vi "Set_Hi-Tec_server.vi"(4 "Client Name":string, 5 "Gas Line Name":T1, 6 "Strength (% by volume)":dbl min=0.0 max=1000.0 format="%.3f", 7 "Carrier_2 Q (l/min)":dbl=20.0 format="%.2f", 8 "Carrier_1 Q (l/min)":dbl=20.0 format="%.2f", 9 "Mode":enum16{"Control Hi-Tec", "Check Hi-Tec Demands"}(ring)) -> (0 "Flowrates (kg/min)":dbl[](array[numeric]) format="%.2f", 1 "Comment":string)   [LabVIEW 2022 SP3]
uses:
  Anemometry/Anemometry Sub Vis/Controls/GMU Gas Line Name.ctl
  ADAM Client/Sub VIs/ADAM Controls/Ch_description_ADAM.ctl
  ADAM Client/Sub VIs/ADAM Controls/Module_type_ADAM.ctl
  ADAM Client/Sub VIs/ADAM Controls/Function_ADAM.ctl
  ADAM Client/Sub VIs/ADAM Controls/Channel_State.ctl
  ADAM Client/Sub VIs/ADAM Controls/Calib_type_ADAM.ctl
  ADAM Client/Sub VIs/ADAM Controls/Address.ctl
  ADAM Client/Sub VIs/ADAM Controls/Update_scan_value.ctl
  Anemometry/Anemometry Sub Vis/Globals/Gas_management_global.vi
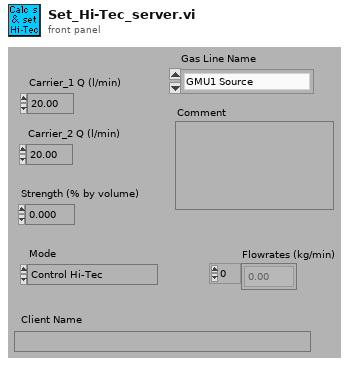
[diagram p1: front panel]
types:
  T1 = typedef "GMU Gas Line Name.ctl" = enum16{"GMU1 Source", "GMU2 Source", "GMU2 Calib", "CPP GRC-A", "CPP GRC-B"}
  T2 = typedef "Module_type_ADAM.ctl" = string
  T3 = typedef "Ch_description_ADAM.ctl" = cluster{"Ch Name":string, "Type":T2, "Function":T4, "Ch State":T5, "Calibration type":T6, "A":dbl, "B":dbl, "C":dbl, "D":dbl, "Comments":string, "Address":T7, "String":string, "Duty":u16}
  T4 = typedef "Function_ADAM.ctl" = enum16{"Analogue Input", "Digital Input", "Event counter", "Event rate", "Analogue Output", "Digital Output", "Relay Output"}
  T5 = typedef "Channel_State.ctl" = enum16{"On", "Off", "Always On", "Always Off"}
  T6 = typedef "Calib_type_ADAM.ctl" = string
  T7 = typedef "Address.ctl" = cluster{"Main":i32, "Ch.":i32, "Sub":i32, "Port Name":string}
  T8 = enum16{"Append to Global", "Read Global then Clear"}
  T9 = typedef "Update_scan_value.ctl" = cluster{"Channel Name":string, "New Value":dbl, "!Auto_Off":bool}
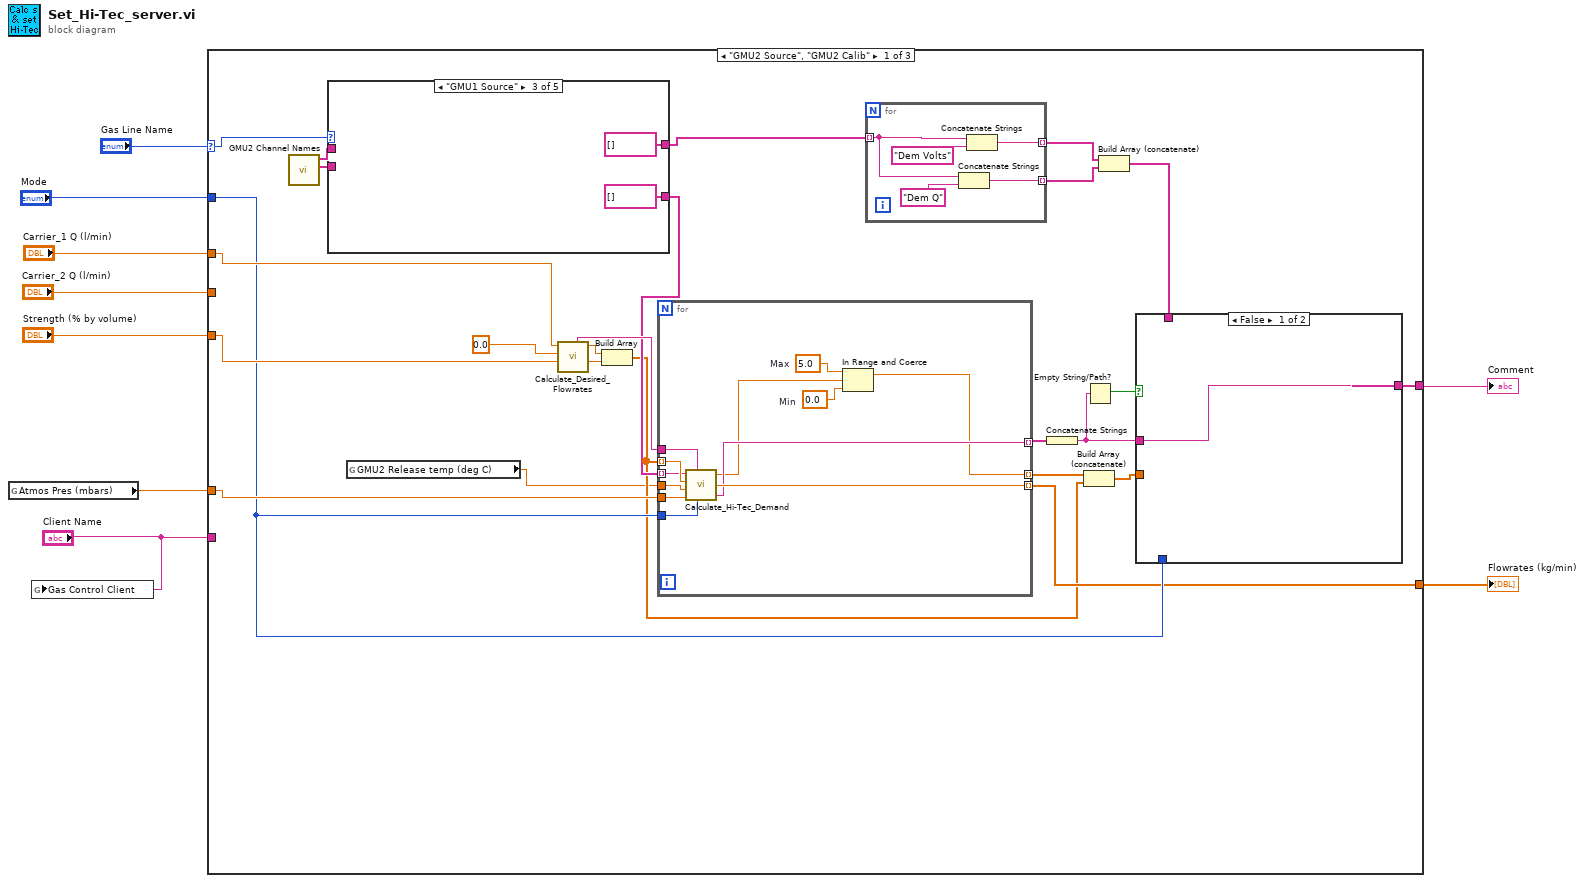
[diagram p0: block diagram]
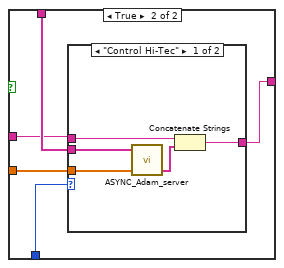
[diagram p2: hidden frame]
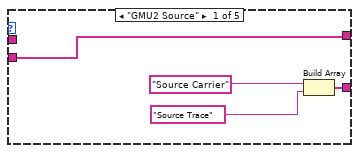
[diagram p4: hidden frame]
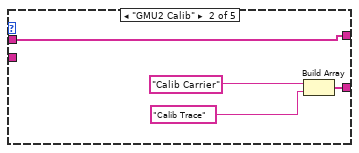
[diagram p5: hidden frame]
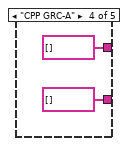
[diagram p6: hidden frame]
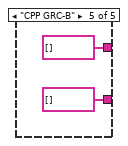
[diagram p7: hidden frame]
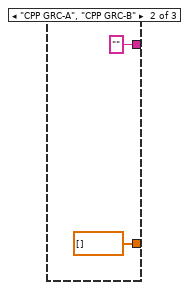
[diagram p8: hidden frame]
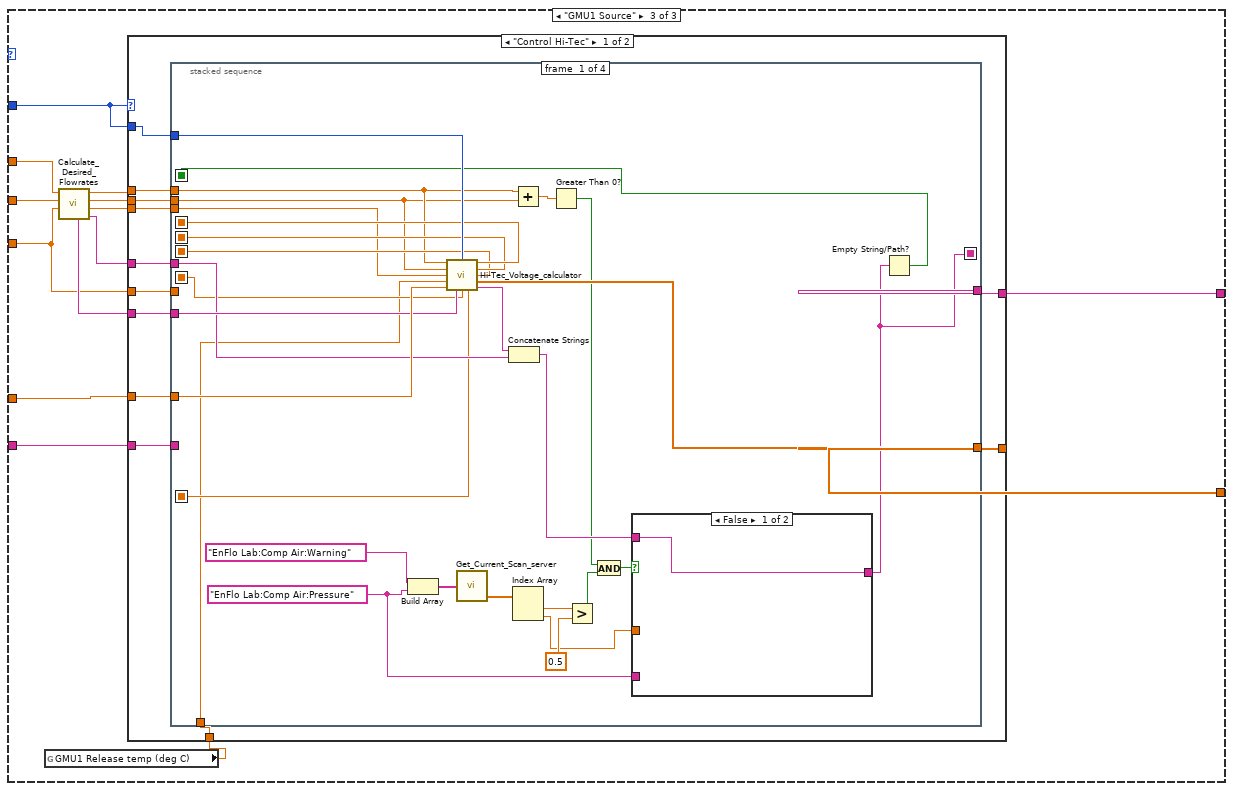
[diagram p9: hidden frame]
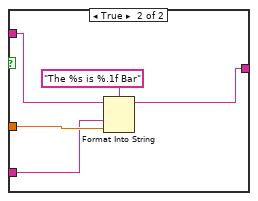
[diagram p10: hidden frame]
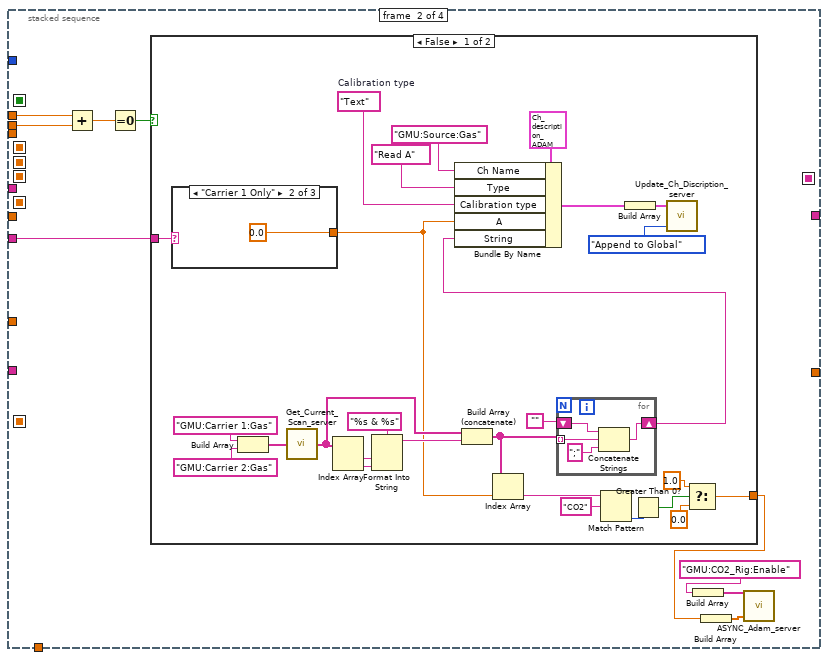
[diagram p11: hidden frame]
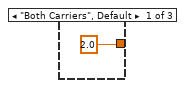
[diagram p12: hidden frame]
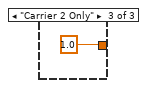
[diagram p13: hidden frame]
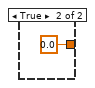
[diagram p14: hidden frame]
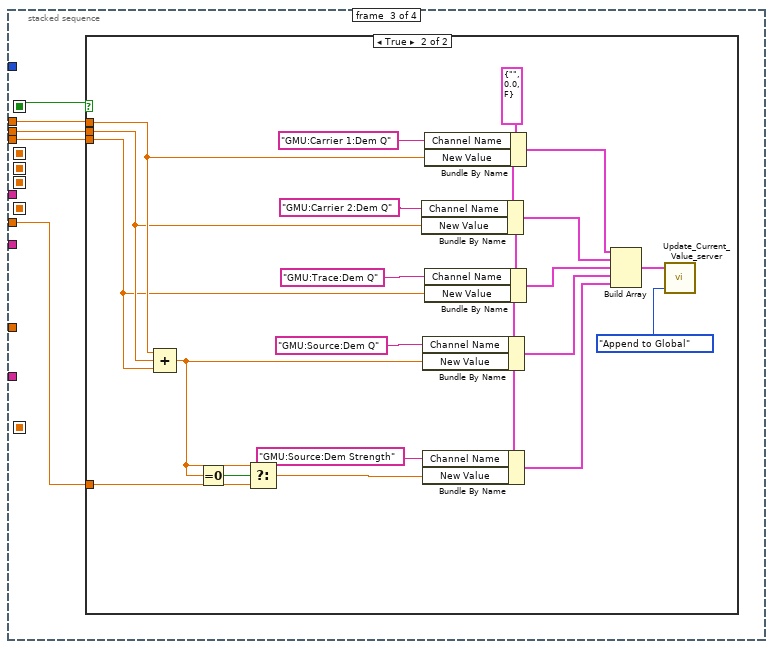
[diagram p15: hidden frame]
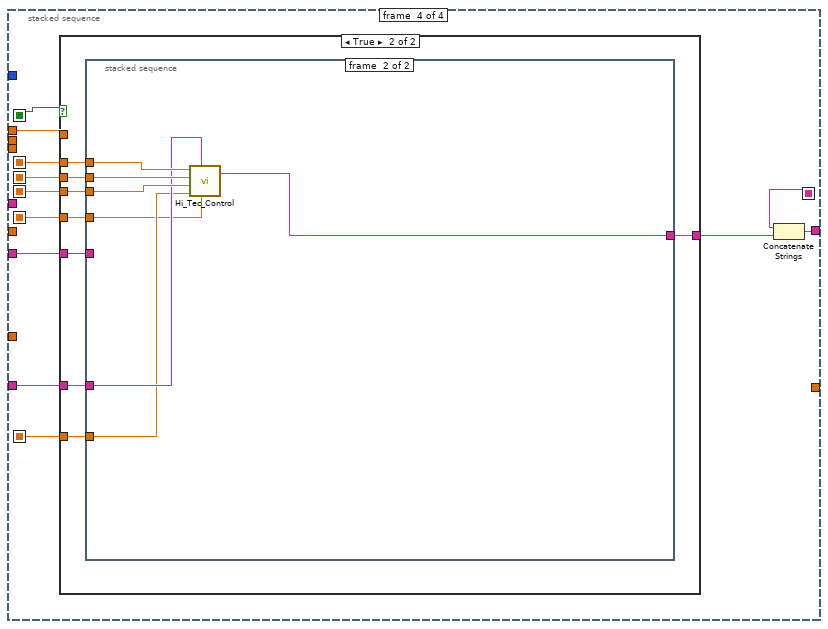
[diagram p17: hidden frame]
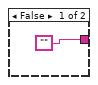
[diagram p18: hidden frame]
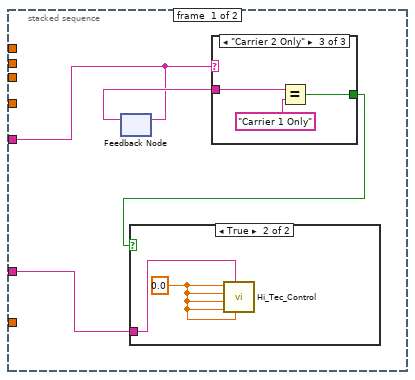
[diagram p19: hidden frame]
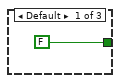
[diagram p20: hidden frame]
diagram:
  n1 = global read "Gas_management_global.vi" "Atmos Pres (mbars)"() -> (w9:dbl)
  n2 = global write "Gas_management_global.vi" "Gas Control Client"("Client Name") -> ()
  n3 = case shown="\"GMU2 Source\", \"GMU2 Calib\"" "Gas Line Name" {
    selector: "Gas Line Name" -> [w27 _ _]
    tunnel: w9 -> [w26 _ w93]
    tunnel: [w24 dbl[] [] ("Flowrates (kg/min)") w92] -> w8
    tunnel: "Mode" -> [w25 _ w91]
    tunnel: "Client Name" -> [_ _ w90]
    tunnel: "Carrier_1 Q (l/min)" -> [w29 _ w89]
    tunnel: "Carrier_2 Q (l/min)" -> [_ _ w88]
    tunnel: "Strength (% by volume)" -> [w28 _ w83]
    tunnel: [w23 "" w81] -> w2
    frame "GMU2 Source", "GMU2 Calib" {
      n4 = call "GMU2 Channel Names.vi"() -> ("GMU2 Source Channels"=w18:string[], "GMU2 Calib Channels"=w11:string[])  [unwired: 10 in]
      n5 = case shown="\"GMU1 Source\"" w27 {
        tunnel: [w55 w59 string[] [] string[] [] string[] []] -> w30
        tunnel: [w52 w56 string[] [] string[] [] ("GMU2 Calib Channels") string[] [] ("GMU2 Calib Channels")] -> w19
        tunnel: w18 -> [w52 _ _ _ _]
        tunnel: w11 -> [_ w56 _ _ _]
        frame "GMU2 Source" {
          n6 = Build Array("Source Carrier", "Source Trace") -> (w55:string[])
        }
        frame "GMU2 Calib" {
          n7 = Build Array("Calib Carrier", "Calib Trace") -> (w59:string[])
        }
        frame "GMU1 Source" {
        }
        frame "CPP GRC-A" {
        }
        frame "CPP GRC-B" {
        }
      }
      n8 = global read "Gas_management_global.vi" "GMU2 Release temp (deg C)"() -> (w10:dbl)
      n9 = call "Calculate_Desired_Flowrates.vi"("Strength (% by volume)"=w28, "Carrier_2 Q (l/min)"=0.0, "Carrier_1 Q (l/min)"=w29) -> ("Trace Q l/min"=w33:dbl, "Carrier 1 l/min"=w34:dbl, "Carrier Info"=w32:string)  [unwired: 3 in, 2 out]
      n10 = Build Array(w34, w33) -> (w12:dbl[])
      n11 = for {
        tunnel: w26 -> [w77]
        tunnel: w10 -> [w76]
        tunnel: w12 -> [w75] mode=indexing
        tunnel: [w72] -> w24 mode=indexing
        tunnel: w30 -> [w74] mode=indexing
        tunnel: w32 -> [w73]
        tunnel: [w66] -> w14 mode=indexing
        tunnel: [w71] -> w22 mode=indexing
        tunnel: w25 -> [w70]
        w68 = 0.0  # Min
        w69 = 5.0  # Max
        n12 = call "Calculate_Hi-Tec_Demand.vi"("Gas Line Name"=w74, "Carrier Info"=w73, "Flowrate"=w75, "Release temp (deg C)"=w76, "Mode"=w70, "Atmos Pres (mbars)"=w77) -> ("Demand Voltage"=w67:dbl, "Flowrate (kg/min)"=w72:dbl, "Error messages"=w71:string)
        n13 = In Range and Coerce(upper limit=w69, x=w67, lower limit=w68) -> (coerced(x)=w66:dbl)  [unwired: 1 out]
      }
      n14 = for {
        tunnel: w19 -> [w37] mode=indexing
        tunnel: [w36] -> w17 mode=indexing
        tunnel: [w35] -> w16 mode=indexing
        n15 = Concatenate Strings(w37, "Dem Q" ("string")) -> (w35:string)
        n16 = Concatenate Strings(w37, "Dem Volts" ("string")) -> (w36:string)
      }
      n17 = Concatenate Strings(w22) -> (w21:string)
      n18 = Build Array (concatenate)(w14, w12) -> (w13:dbl[])
      n19 = Empty String/Path?(string/path=w21) -> (empty?=w20:bool)
      n20 = Build Array (concatenate)(w17, w16) -> (w15:string[])
      n21 = case shown="False" w20 {
        tunnel: w15 -> [_ w45]
        tunnel: w13 -> [_ w44]
        tunnel: w25 -> [_ w43]
        tunnel: [w40 w42] -> w23
        tunnel: w21 -> [w40 w41]
        frame False {
        }
        frame True {
          n22 = case shown="\"Control Hi-Tec\"" w43 {
            tunnel: w45 -> [w50 _]
            tunnel: w44 -> [w49 _]
            tunnel: w41 -> [w47 w51]
            tunnel: [w46 w51] -> w42
            frame "Control Hi-Tec" {
              n23 = call "ASYNC_Adam_server.vi"("Values"=w49, "Channel Names"=w50) -> ("Scan Comments"=w48:string[])  [unwired: 1 in, 2 out]
              n24 = Concatenate Strings(w47, w48) -> (w46:string)
            }
            frame "Check Hi-Tec Demands" {
            }
          }
        }
      }
    }
    frame "CPP GRC-A", "CPP GRC-B" {
    }
    frame "GMU1 Source" {
      n25 = global read "Gas_management_global.vi" "GMU1 Release temp (deg C)"() -> (w80:dbl)
      n26 = call "Calculate_Desired_Flowrates.vi"("Strength (% by volume)"=w83, "Carrier_2 Q (l/min)"=w88, "Carrier_1 Q (l/min)"=w89) -> ("Error Message"=w82:string, "Trace Q l/min"=w85:dbl, "Carrier 2 l/min"=w86:dbl, "Carrier 1 l/min"=w87:dbl, "Carrier Info"=w84:string)  [unwired: 3 in]
      n27 = case shown="\"Control Hi-Tec\"" w91 {
        tunnel: w87 -> [w105 w260]
        tunnel: w93 -> [w104 w261]
        tunnel: [w103 w253] -> w81
        tunnel: [w102 w259] -> w92
        tunnel: w91 -> [w101 w258]
        tunnel: w90 -> [w100 _]
        tunnel: w86 -> [w99 w257]
        tunnel: w85 -> [w98 w256]
        tunnel: w84 -> [w97 w255]
        tunnel: w83 -> [w96 _]
        tunnel: w82 -> [w95 w252]
        tunnel: w80 -> [w94 w251]
        frame "Control Hi-Tec" {
          n28 = stacked-sequence {
            seq-local: [w132 _ _ _] -> [_ _ w189 w217]
            seq-local: [w131 _ _ _] -> [_ _ _ w221]
            seq-local: [w130 _ _ _] -> [_ _ _ w220]
            seq-local: [w129 _ _ _] -> [_ _ _ w219]
            seq-local: [w116 _ _ _] -> [_ _ _ w214]
            seq-local: [w123 _ _ _] -> [_ _ _ w211]
            seq-local: [w122 _ _ _] -> [_ _ _ w210]
            tunnel: w99 -> [w112 w141 w187 _]
            tunnel: w105 -> [w113 w142 w188 w216]
            tunnel: w104 -> [w134 _ _ _]
            tunnel: [_ _ _ w215] -> w103
            tunnel: [w126 _ _ _] -> w102
            tunnel: w101 -> [w133 _ _ _]
            tunnel: w100 -> [_ _ _ w218]
            tunnel: w98 -> [w128 _ w186 _]
            tunnel: w97 -> [w127 w144 _ w212]
            tunnel: w96 -> [_ _ w185 _]
            tunnel: w95 -> [w124 _ _ _]
            tunnel: w94 -> [w106 _ _ _]
            frame #0 {
              w107 = "EnFlo Lab:Comp Air:Pressure"
              n29 = Build Array("EnFlo Lab:Comp Air:Warning", w107) -> (w121:string[])
              n30 = call "Hi-Tec_Voltage_calculator.vi"("Carrier_1 Q (l/min)"=w113, "Mode"=w133, "Carrier_2 Q (l/min)"=w112, "Trace Q (l/min)"=w128, "Release temp (deg C)"=w106, "Atmos Pres (mbars)"=w134, "Carrier Info"=w127) -> ("Carrier 1 Voltage"=w131:dbl, "Carrier 2 Voltage"=w130:dbl, "Trace Voltage"=w129:dbl, "Flowrates (kg/min)"=w126:dbl[], "Carrier 1_50 Voltage"=w122:dbl, "Trace_2 Voltage"=w123:dbl, "Error Comments"=w125:string)  [unwired: 1 in, 1 out]
              n31 = call "Get_Current_Scan_server.vi"("Desired Channels"=w121) -> ("Numerical Values"=w119:dbl[])  [unwired: 2 out]
              n32 = Concatenate Strings(w125, w124) -> (w115:string)
              n33 = Add(x=w113, y=w112) -> (x+y=w114:dbl)
              n34 = Index Array(array=w119) -> (element #1=w118:dbl, element #2=w108:dbl)  [unwired: 2 in]
              n35 = Greater Than 0?(x=w114) -> (x > 0?=w110:bool)
              n36 = Greater?(x=w118, y=0.5) -> (0:w111:bool)
              n37 = And(x=w110, y=w111) -> (x .and. y?=w109:bool)
              n38 = case shown="False" w109 {
                tunnel: [w135 w136] -> w116
                tunnel: w115 -> [w135 w139]
                tunnel: w108 -> [_ w140]
                tunnel: w107 -> [_ w137]
                frame False {
                }
                frame True {
                  n39 = Format Into String(format string="The %s is %.1f Bar", initial string=w139, w137, w140) -> (resulting string=w136:string)  [unwired: 1 in, 1 out]
                }
              }
              n40 = Empty String/Path?(string/path=w116) -> (empty?=w132:bool)
            }
            frame #1 {
              n41 = Add(x=w142, y=w141) -> (x+y=w143:dbl)
              n42 = Equal To 0?(x=w143) -> (x = 0?=w149:bool)
              n43 = case shown="False" w149 {
                tunnel: w144 -> [w175 _]
                tunnel: [w151 0.0 ("f")] -> w145
                frame False {
                  w150 = T6 "Text"  # Calibration type
                  n44 = case shown="\"Carrier 1 Only\"" w175 {
                    tunnel: [2.0 ("A") 0.0 ("A") 1.0 ("A")] -> w158
                    frame "Both Carriers", Default {
                    }
                    frame "Carrier 1 Only" {
                    }
                    frame "Carrier 2 Only" {
                    }
                  }
                  n45 = Build Array("GMU:Carrier 1:Gas", "GMU:Carrier 2:Gas") -> (w174:string[])
                  n46 = call "Get_Current_Scan_server.vi"("Desired Channels"=w174) -> ("String values"=w164:string[])  [unwired: 2 out]
                  n47 = Index Array(array=w164) -> (element #1=w167:string, element #2=w166:string)  [unwired: 2 in]
                  n48 = Format Into String(format string="%s & %s", w167, w166) -> (resulting string=w163:string)  [unwired: 2 in, 1 out]
                  n49 = Build Array (concatenate)(w164, w163) -> (w159:string[])
                  n50 = Index Array(array=w159, index=w158) -> (element=w156:string)
                  n51 = for {
                    shift-right: [w180] -> w160
                    shift-left: "" -> [w179]
                    tunnel: w159 -> [w178] mode=indexing
                    n52 = Concatenate Strings(w179, w178, ";" ("string")) -> (w180:string)
                  }
                  n53 = Bundle By Name(cluster=T3 {"Ch Name"="", "Type"="", "Function"=enum."Analogue Input", "Ch State"=enum."On", "Calibration type"="", "A"=0.0, "B"=0.0, "C"=0.0, "D"=0.0, "Comments"="", "Address"={"Main"=0, "Ch."=0, "Sub"=0, "Port Name"=""}, "String"="", "Duty"=65535} ("Ch Discription"), "Ch Name"="GMU:Source:Gas", "Type"=T2 "Read A", "Calibration type"=w150, "A"=w158, "String"=w160) -> (w169:T3)
                  n54 = Match Pattern(string=w156, regular expression="CO2") -> (offset past match=w155:i32)  [unwired: 1 in, 3 out]
                  n55 = Build Array(w169) -> (w176:T3[])
                  n56 = Greater Than 0?(x=w155) -> (x > 0?=w154:bool)
                  n57 = call "Update_Ch_Discription_server.vi"("Mode"=T8."Append to Global", "Channels to update In"=w176) -> ()  [unwired: 1 in, 1 out]
                  n58 = Select(t=1.0, s=w154, f=0.0) -> (s? t:f=w151:dbl)
                }
                frame True {
                }
              }
              n59 = Build Array("GMU:CO2_Rig:Enable") -> (w147:string[])
              n60 = Build Array(w145) -> (w148:dbl[])
              n61 = call "ASYNC_Adam_server.vi"("Values"=w148, "Channel Names"=w147) -> ()  [unwired: 1 in, 3 out]
            }
            frame #2 {
              n62 = case shown="True" w189 {
                tunnel: w188 -> [_ w200]
                tunnel: w187 -> [_ w199]
                tunnel: w186 -> [_ w198]
                tunnel: w185 -> [_ w196]
                frame False {
                }
                frame True {
                  w195 = T9 {"Channel Name"="", "New Value"=0.0, "!Auto_Off"=FALSE} ("Update Scan Value Cluster")
                  n63 = Compound Arithmetic op=ADD(w200, w199, w198) -> (w197:dbl)
                  n64 = Equal To 0?(x=w197) -> (x = 0?=w205:bool)
                  n65 = Select(t=w197, s=w205, f=w196) -> (s? t:f=w204:dbl)
                  n66 = Bundle By Name(cluster=w195, "Channel Name"="GMU:Carrier 2:Dem Q", "New Value"=w199) -> (w193:T9)
                  n67 = Bundle By Name(cluster=w195, "Channel Name"="GMU:Source:Dem Q", "New Value"=w197) -> (w191:T9)
                  n68 = Bundle By Name(cluster=w195, "Channel Name"="GMU:Source:Dem Strength", "New Value"=w204) -> (w190:T9)
                  n69 = Bundle By Name(cluster=w195, "Channel Name"="GMU:Carrier 1:Dem Q", "New Value"=w200) -> (w194:T9)
                  n70 = Bundle By Name(cluster=w195, "Channel Name"="GMU:Trace:Dem Q", "New Value"=w198) -> (w192:T9)
                  n71 = Build Array(w194, w193, w192, w191, w190) -> (w207:T9[])
                  n72 = call "Update_Current_Value_server.vi"("Mode"=T8."Append to Global", "Update array in"=w207) -> ()  [unwired: 1 in, 1 out]
                }
              }
            }
            frame #3 {
              n73 = case shown="True" w217 {
                tunnel: w221 -> [_ w230]
                tunnel: w220 -> [_ w229]
                tunnel: w219 -> [_ w228]
                tunnel: w218 -> [_ w227]
                tunnel: w216 -> [_ _]
                tunnel: ["" w226] -> w213
                tunnel: w212 -> [_ w225]
                tunnel: w211 -> [_ w224]
                tunnel: w210 -> [_ w223]
                frame False {
                }
                frame True {
                  n74 = stacked-sequence {
                    tunnel: w230 -> [_ w250]
                    tunnel: w229 -> [_ w249]
                    tunnel: w228 -> [_ w248]
                    tunnel: w227 -> [w234 w247]
                    tunnel: [_ w246] -> w226
                    tunnel: w225 -> [w231 _]
                    tunnel: w224 -> [_ w245]
                    tunnel: w223 -> [_ w244]
                    frame #0 {
                      n75 = feedback-in #1(w231) -> ()
                      n76 = feedback #1() -> (w233:string)  [unwired: 1 in]
                      n77 = case shown="\"Carrier 2 Only\"" w231 {
                        tunnel: w233 -> [_ w238 w241]
                        tunnel: [FALSE w236 w239] -> w232
                        frame Default {
                        }
                        frame "Carrier 1 Only" {
                          n78 = Equal?(x=w238, y="Carrier 2 Only") -> (x = y?=w236:bool)
                        }
                        frame "Carrier 2 Only" {
                          n79 = Equal?(x=w241, y="Carrier 1 Only") -> (x = y?=w239:bool)
                        }
                      }
                      n80 = case shown="True" w232 {
                        tunnel: w234 -> [_ w243]
                        frame False {
                        }
                        frame True {
                          w242 = 0.0 ("Carrier 1 Voltage")
                          n81 = call "Hi_Tec_Control.vi"("Carrier 1_50 Voltage"=w242, "Client Name"=w243, "Trace_2 Voltage"=w242, "Trace Voltage"=w242, "Carrier 2 Voltage"=w242, "Carrier 1 Voltage"=w242) -> ()  [unwired: 1 in, 1 out]
                        }
                      }
                    }
                    frame #1 {
                      n82 = call "Hi_Tec_Control.vi"("Carrier 1_50 Voltage"=w244, "Client Name"=w247, "Trace_2 Voltage"=w245, "Trace Voltage"=w248, "Carrier 2 Voltage"=w249, "Carrier 1 Voltage"=w250) -> ("Scan Comments"=w246:string)  [unwired: 1 in]
                    }
                  }
                }
              }
              n83 = Concatenate Strings(w214, w213) -> (w215:string)
            }
          }
        }
        frame "Check Hi-Tec Demands" {
          n84 = call "Hi-Tec_Voltage_calculator.vi"("Carrier_1 Q (l/min)"=w260, "Mode"=w258, "Carrier_2 Q (l/min)"=w257, "Trace Q (l/min)"=w256, "Release temp (deg C)"=w251, "Atmos Pres (mbars)"=w261, "Carrier Info"=w255) -> ("Flowrates (kg/min)"=w259:dbl[], "Error Comments"=w254:string)  [unwired: 1 in, 6 out]
          n85 = Concatenate Strings(w254, w252) -> (w253:string)
        }
      }
    }
  }
  "Comment" <- w2
  "Flowrates (kg/min)" <- w8
